vi "Log Test Results and Data.vi"(0 "Test Results in in":T1, 11 "error in (no error)":errorcluster) -> (15 "error out":errorcluster)   [LabVIEW 2016]
doc: "This VI saves test report and test data to log files."
uses:
  controls/Test Results.ctl
  <vilib>/Utility/file.llb/Write To Spreadsheet File (string).vi
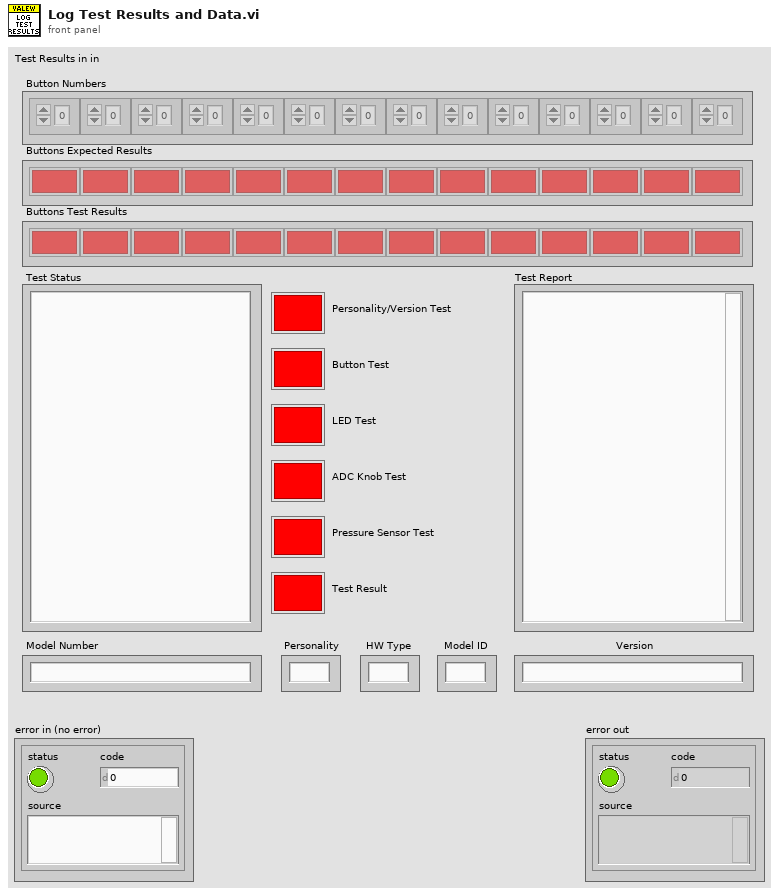
[diagram p1: front panel]
types:
  T1 = typedef "Test Results.ctl" = cluster{"Test Status":string, "Personality/Version Test ":bool, "Test Report":string, "Model Number":string, "Button Numbers":i32[], "Buttons Test Results":bool[], "Buttons Expected Results":bool[], "Model ID":string, "Personality":string, "HW Type":string, "Version":string, "Button Test":bool, "LED Test":bool, "ADC Knob Test":bool, "Pressure Sensor Test":bool, "Test Result":bool}
  T2 = enum16{"open", "replace", "create", "open or create", "replace or create", "replace or create with confirmation"}
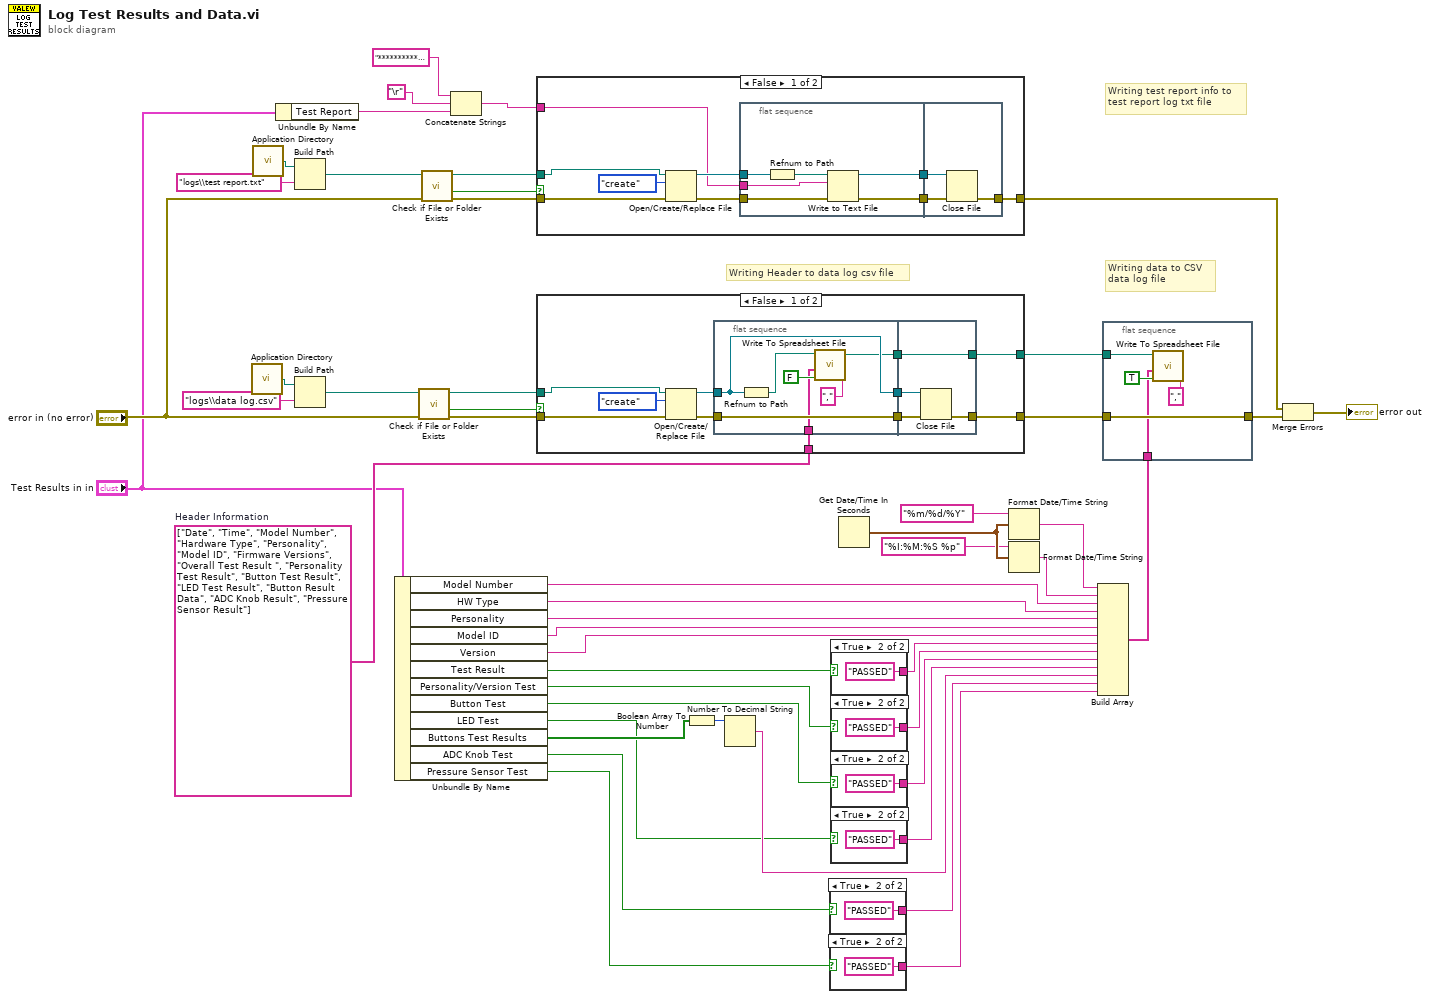
[diagram p0: block diagram]
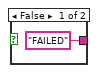
[diagram p2: hidden frame]
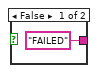
[diagram p3: hidden frame]
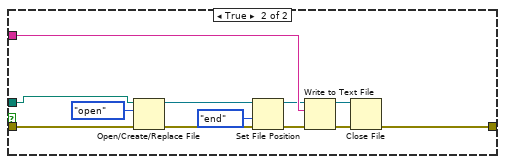
[diagram p4: hidden frame]
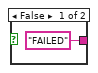
[diagram p5: hidden frame]
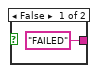
[diagram p6: hidden frame]
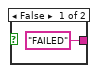
[diagram p7: hidden frame]
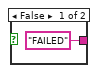
[diagram p8: hidden frame]
diagram:
  w33 = string[] ["Date", "Time", "Model Number", "Hardware Type", "Personality", "Model ID", "Firmware Versions", "Overall Test Result ", "Personality Test Result", "Button Test Result", "LED Test Result", "Button Result Data", "ADC Knob Result", "Pressure Sensor Result"]  # Header Information
  # "Writing Header to data log csv file"
  # "Writing test report info to \ntest report log txt file"
  # "Writing data to CSV \ndata log file"
  n1 = call <vilib>:"Application Directory.vi"() -> ("Application Directory"=w27:path)
  n2 = call <vilib>:"Application Directory.vi"() -> ("Application Directory"=w24:path)
  n3 = Unbundle By Name("Test Results in in") -> ("Test Report"=w13:string)
  n4 = Build Path(base path=w24, name or relative path="logs\\test report.txt") -> (appended path=w23:path)
  n5 = Build Path(base path=w27, name or relative path="logs\\data log.csv") -> (appended path=w29:path)
  n6 = Unbundle By Name("Test Results in in") -> ("Model Number"=w40:string, "HW Type"=w41:string, "Personality"=w9:string, "Model ID"=w8:string, "Version"=w5:string, "Test Result"=w7:bool, "Personality/Version Test"=w48:bool, "Button Test"=w49:bool, "LED Test"=w10:bool, "Buttons Test Results"=w46:bool[], "ADC Knob Test"=w4:bool, "Pressure Sensor Test"=w3:bool)
  n7 = call <vilib>:"Check if File or Folder Exists.vi"("error in (no error)"="error in (no error)", "path"=w29) -> ("error out"=w30:errorcluster, "file or folder exists?"=w32:bool, "dup path"=w31:path)  [unwired: 7 in]
  n8 = call <vilib>:"Check if File or Folder Exists.vi"("error in (no error)"="error in (no error)", "path"=w23) -> ("error out"=w22:errorcluster, "file or folder exists?"=w20:bool, "dup path"=w21:path)  [unwired: 7 in]
  n9 = Concatenate Strings("***********************************************************************************************", "\r", w13) -> (w14:string)
  n10 = case shown="False" w20 {
    tunnel: w21 -> [w56 w70]
    tunnel: w22 -> [w58 w76]
    tunnel: [w55 w79] -> w16
    tunnel: w14 -> [w51 w78]
    frame False {
      n11 = Open/Create/Replace File(file path (use dialog)=w56, error in=w58, operation (0:open)=T2."create") -> (refnum out=w53:refnum<file>, error out=w57:errorcluster)  [unwired: 3 in, 1 out]
      n12 = flat-sequence {
        tunnel: w57 -> [w65]
        tunnel: [w64] -> w54
        tunnel: w53 -> [w61]
        tunnel: [w60] -> w52
        tunnel: w51 -> [w62]
        tunnel: [w67] -> w55
        tunnel: w54 -> [w68]
        tunnel: w52 -> [w66]
        frame #0 {
          n13 = Refnum to Path(1:w61) -> (0:w63:path)
          n14 = Write to Text File(file (use dialog)=w63, text=w62, error in=w65) -> (refnum out=w60:refnum<file>, error out=w64:errorcluster)  [unwired: 1 in, 1 out]
        }
        frame #1 {
          n15 = Close File(refnum=w66, error in=w68) -> (error out=w67:errorcluster)  [unwired: 1 out]
        }
      }
    }
    frame True {
      n16 = Open/Create/Replace File(file path (use dialog)=w70, error in=w76, operation (0:open)=T2."open") -> (refnum out=w69:refnum<file>, error out=w72:errorcluster)  [unwired: 3 in, 1 out]
      n17 = Set File Position(refnum=w69, from (0:start)=enum16{"start", "end", "current"}."end", error in=w72) -> (refnum out=w74:refnum<file>, error out=w75:errorcluster)  [unwired: 1 in]
      n18 = Write to Text File(file (use dialog)=w74, text=w78, error in=w75) -> (refnum out=w77:refnum<file>, error out=w80:errorcluster)  [unwired: 1 in, 1 out]
      n19 = Close File(refnum=w77, error in=w80) -> (error out=w79:errorcluster)  [unwired: 1 out]
    }
  }
  n20 = case shown="False" w32 {
    tunnel: w31 -> [w88 w104]
    tunnel: [w81 w104] -> w28
    tunnel: w30 -> [w90 w103]
    tunnel: [w87 w103] -> w34
    tunnel: w33 -> [w84 _]
    frame False {
      n21 = Open/Create/Replace File(file path (use dialog)=w88, error in=w90, operation (0:open)=T2."create") -> (refnum out=w85:refnum<file>, error out=w89:errorcluster)  [unwired: 3 in, 1 out]
      n22 = flat-sequence {
        tunnel: w89 -> [w98]
        tunnel: [w98] -> w86
        tunnel: w85 -> [w93]
        tunnel: w84 -> [w94]
        tunnel: [w93] -> w83
        tunnel: [w92] -> w82
        tunnel: [w101] -> w87
        tunnel: w86 -> [w102]
        tunnel: w83 -> [w100]
        tunnel: [w99] -> w81
        tunnel: w82 -> [w99]
        frame #0 {
          n23 = Refnum to Path(1:w93) -> (0:w97:path)
          n24 = call-poly <vilib>:"Write To Spreadsheet File.vi"("delimiter (\\t)"=",", "append to file? (new file:F)"=FALSE, "1D data"=w94, "file path (dialog if empty)"=w97) -> ("new file path (Not A Path if cancelled)"=w92:path)  [unwired: 4 in]
        }
        frame #1 {
          n25 = Close File(refnum=w100, error in=w102) -> (error out=w101:errorcluster)  [unwired: 1 out]
        }
      }
    }
    frame True {
    }
  }
  n26 = Boolean Array To Number(Boolean array=w46) -> (number=w45:u32)
  n27 = Number To Decimal String(number=w45) -> (decimal integer string=w50:string)  [unwired: 1 in]
  n28 = case shown="True" w4 {
    tunnel: ["FAILED" "PASSED"] -> w2
    frame False {
    }
    frame True {
    }
  }
  n29 = case shown="True" w3 {
    tunnel: ["FAILED" "PASSED"] -> w1
    frame False {
    }
    frame True {
    }
  }
  n30 = case shown="True" w7 {
    tunnel: ["FAILED" "PASSED"] -> w6
    frame False {
    }
    frame True {
    }
  }
  n31 = case shown="True" w48 {
    tunnel: ["FAILED" "PASSED"] -> w42
    frame False {
    }
    frame True {
    }
  }
  n32 = case shown="True" w49 {
    tunnel: ["FAILED" "PASSED"] -> w43
    frame False {
    }
    frame True {
    }
  }
  n33 = case shown="True" w10 {
    tunnel: ["FAILED" "PASSED"] -> w44
    frame False {
    }
    frame True {
    }
  }
  n34 = Get Date/Time In Seconds() -> (seconds since 1Jan1904=w37:timestamp)
  n35 = Format Date/Time String(time format string (%c)="%m/%d/%Y", seconds (now)=w37) -> (date/time string=w38:string)  [unwired: 1 in]
  n36 = Format Date/Time String(time format string (%c)="%I:%M:%S %p", seconds (now)=w37) -> (date/time string=w39:string)  [unwired: 1 in]
  n37 = Build Array(w38, w39, w40, w41, w9, w8, w5, w6, w42, w43, w44, w50, w2, w1) -> (w47:string[])
  n38 = flat-sequence {
    tunnel: w28 -> [w121]
    tunnel: [w118] -> w18
    tunnel: w34 -> [w118]
    tunnel: w47 -> [w117]
    frame #0 {
      n39 = call-poly <vilib>:"Write To Spreadsheet File.vi"("delimiter (\\t)"=",", "append to file? (new file:F)"=TRUE, "1D data"=w117, "file path (dialog if empty)"=w121) -> ()  [unwired: 4 in, 1 out]
    }
  }
  n40 = Merge Errors(w16, w18) -> (→"error out":errorcluster)
